vi "EncoderDistance.vi"(3 "Encoder":string="My Encoder RefNum") -> (1 "Encoder Distance":dbl)   [LabVIEW 2014]
doc: "This example shows how to configure, read values from, and reset an encoder.\n\nIt will display the encoder value, period, direction, and if the encoder is stopped.\n\nThis example expects a USB cable connected from your development PC to the Type B USB Jack (next to the power input) on the roboRIO."
panel:
  out "Encoder Rate (distance/sec)":dbl
  in  "stop":bool
  out "Encoder Alarm Status":string
  out "Encoder Direction":string
  # "Set these inputs before running."
  # "This can be set while running."
  # "Output information."
  # "This shows wiring for a generic quadrature encoder.  Some encoders may have Gnd labeled as Com.  Some may have +5V labeled as +VDC."
  # "Encoder\nB (white wire)---------\nGnd (black wire)------\n+5V (red wire)---------\nA (white wire)---------"
  # "roboRIO\nDIO-1  S\nDIO-0 \nDIO-0  V\nDIO-0  S"
  # "Encoder"
  # "Index"
  # "Gnd"
  # "+5V"
  # "B"
  # "A"
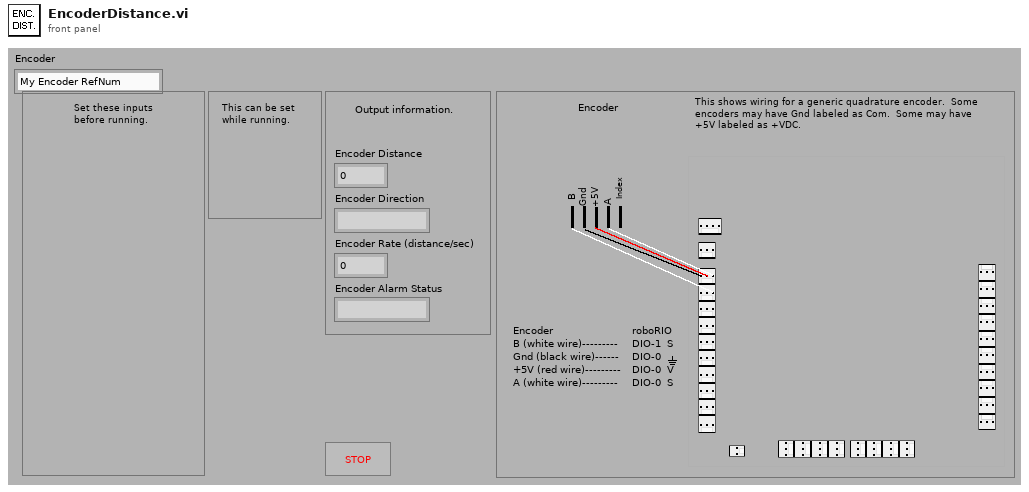
[diagram p1: front panel]
types:
  T1 = typedef "WPI_EncoderDevRef.ctl" = cluster{"DevStatus":errorcluster, "EncoderIndex":T2, "CounterIndex":T3, "DistancePerCount":dbl, "Decoding Type":T4}
  T2 = typedef "FPGA_EncoderIdx.ctl" = enum8{"Enc 0", "Enc 1", "Enc 2", "Enc 3", "Enc 4", "Enc 5", "Enc 6", "Enc 7", "Invalid"}
  T3 = typedef "FPGA_CounterCtrSystemIndex.ctl" = enum8{"Ctr 0", "Ctr 1", "Ctr 2", "Ctr 3", "Ctr 4", "Ctr 5", "Ctr 6", "Ctr 7", "Invalid"}
  T4 = typedef "WPI_EncoderType.ctl" = enum16{"1x", "2x", "4x"}
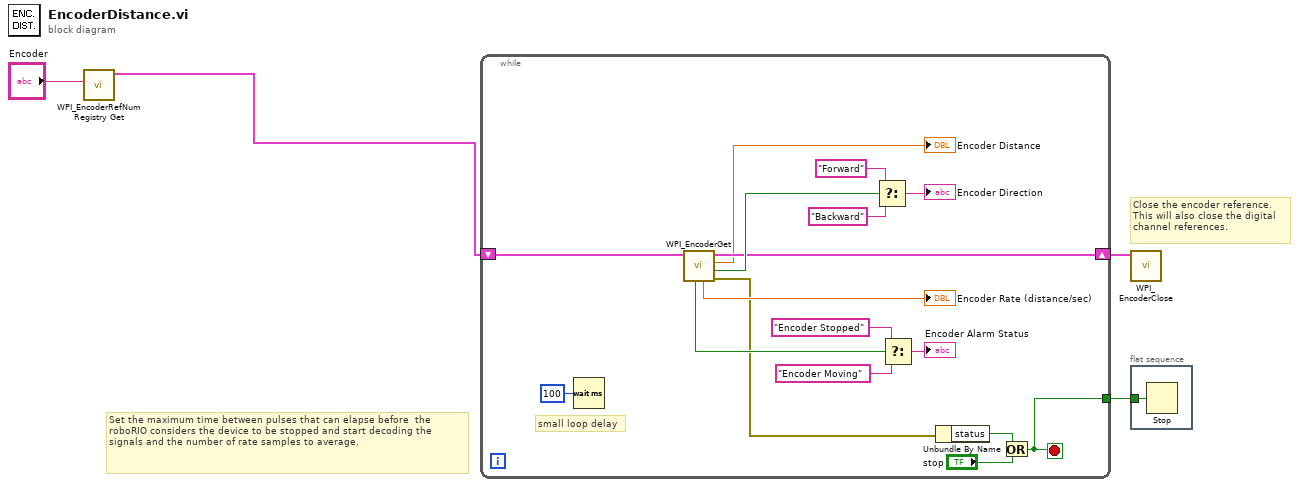
[diagram p0: block diagram]
diagram:
  # "Close the encoder reference.\nThis will also close the digital \nchannel references."
  # "Set the maximum time between pulses that can elapse before  the roboRIO considers the device to be stopped and start decoding the signals and the number of rate samples to average."
  n1 = call <vilib>:"WPI_EncoderRefNum Registry Get.vi"("refnum name"="Encoder") -> ("EncoderDevRef"=w1:T1)  [unwired: 9 in, 1 out]
  n2 = while {
    shift-right: [w16] -> w4
    shift-left: w1 -> [w5]
    tunnel: [w13] -> w3
    stop <- w13 stop-if-true
    # "small loop delay"
    n3 = Wait (ms)(milliseconds to wait=u32 100) -> ()  [unwired: 1 out]
    n4 = call <vilib>:"WPI_EncoderGet.vi"("EncoderDevRef"=w5) -> ("error out"=w12:errorcluster, "Direction"=w18:bool, "Distance"=→"Encoder Distance":dbl, "EncoderDevRef"=w16:T1, "Rate"=→"Encoder Rate (distance/sec)":dbl, "Stopped"=w17:bool)  [unwired: 1 in, 4 out]
    n5 = Select(t="Forward", s=w18, f="Backward") -> (s? t:f=→"Encoder Direction":string)
    n6 = Select(t="Encoder Stopped", s=w17, f="Encoder Moving") -> (s? t:f=→"Encoder Alarm Status":string)
    n7 = Unbundle By Name(w12) -> ("status"=w10:bool)
    n8 = Or(x=w10, y="stop") -> (x .or. y?=w13:bool)
  }
  n9 = call <vilib>:"WPI_EncoderClose.vi"("EncoderDevRef"=w4) -> ()  [unwired: 2 in, 9 out]
  n10 = flat-sequence {
    tunnel: w3 -> [w22]
    frame #0 {
      n11 = Stop(stop? (T)=w22) -> ()
    }
  }
